vi "Module Init.vi"(8 "error in (no error)":errorcluster, 11 "Messaging Server Module in":refnum<class "Messaging Server Module.lvclass">) -> (0 "error out":errorcluster, 3 "Messaging Server Module out":refnum<class "Messaging Server Module.lvclass">)   [LabVIEW 2020, in "Volatus.lvlib" / "Messaging Server Module.lvclass"]
uses:
  Messaging Server Module.lvclass
  Messaging Server Module.lvclass/Messaging Server Module.ctl
  Module/Module.lvclass
  C:/dev/lv20CE/relink/lv-volatus/Volatus/Module/Module.lvclass
  C:/dev/lv20CE/relink/lv-volatus/Volatus/Messaging Server Module/Messaging Server Module.lvclass
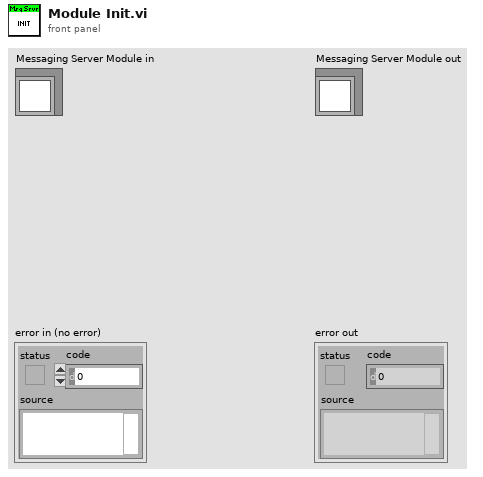
[diagram p1: front panel]
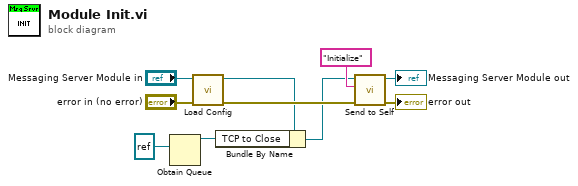
[diagram p0: block diagram]
diagram:
  n1 = Obtain Queue(element data type=refnum<k5> refnum ("TCP Network Connection Refnum")) -> (queue out=w3:refnum<queue>)  [unwired: 4 in, 2 out]
  n2 = call "Load Config.vi"("error in (no error)"="error in (no error)", "Messaging Server Module in"="Messaging Server Module in") -> ("error out"=w9:errorcluster, "Messaging Server Module out"=w2:refnum<class "Messaging Server Module.lvclass">)  [unwired: 8 in]
  n3 = Bundle By Name(cluster=w2, "TCP to Close"=w3) -> (w1:refnum<class "Messaging Server Module.lvclass">)
  n4 = call "Send to Self.vi"("error in (no error)"=w9, "Message ID"="Initialize", "Module in"=w1) -> ("error out"=→"error out":errorcluster, "Module out"=→"Messaging Server Module out":refnum<class "Messaging Server Module.lvclass">)  [unwired: 7 in]
